vi "Wveform grapg break_0.vi"() -> ()   [LabVIEW 2015]
uses:
  <vilib>/measure/NI_MABase.lvlib
panel:
  in  "stop":bool
  in  "Tab Control":enum32{"Page 1"}(tab)
  out "Waveform Graph 2":waveform(dbl)(graph)
  out "Waveform Graph":waveform(dbl)(graph)
  # "Waveform function palette\nwaveform graph break"
  # "Pardeep Kumar"
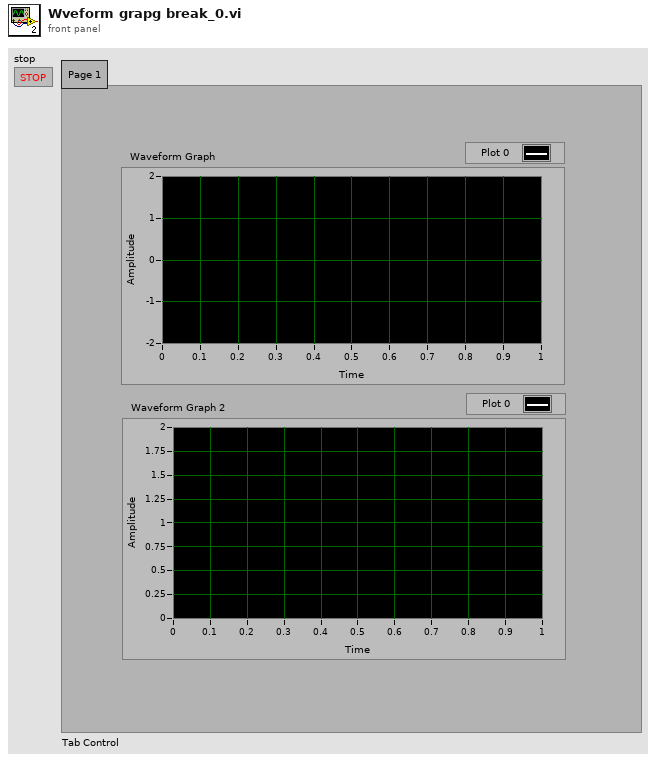
[diagram p1: front panel]
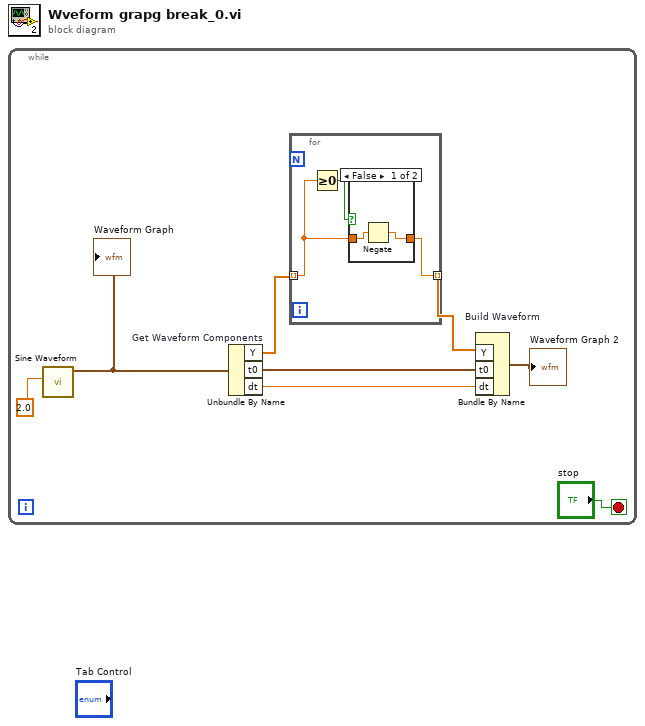
[diagram p0: block diagram]
diagram:
  n1 = while {
    stop <- "stop" stop-if-true
    n2 = call <vilib>:"Sine Waveform.vi"("amplitude"=2.0) -> ("signal out"=w8:waveform(dbl))  [unwired: 9 in, 1 out]
    "Waveform Graph" <- w8
    n3 = Unbundle By Name "Get Waveform Components"(w8) -> ("Y"=w7:dbl[], "t0"=w5:timestamp, "dt"=w4:dbl)
    n4 = for {
      tunnel: w7 -> [w10] mode=indexing
      tunnel: [w9] -> w6 mode=indexing
      n5 = Greater Or Equal To 0?(x=w10) -> (x >= 0?=w11:bool)
      n6 = case shown="False" w11 {
        tunnel: w10 -> [w13 w14]
        tunnel: [w12 w14] -> w9
        frame False {
          n7 = Negate(x=w13) -> (-x=w12:dbl)
        }
        frame True {
        }
      }
    }
    n8 = Bundle By Name "Build Waveform"("Y"=w6, "t0"=w5, "dt"=w4) -> (→"Waveform Graph 2":waveform(dbl))  [unwired: 1 in]
  }
